vi "Mean Selected.vi"(11 "Mean Data":dbl[](array[numeric])) -> (3 "mean":dbl)   [LabVIEW 2020]
uses:
  <vilib>/Analysis/NI_AALBase.lvlib
  <vilib>/Analysis/baseanly.llb/Mean (DBL).vi
  PCT FGV CMD.ctl
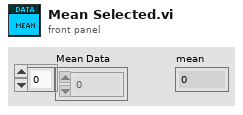
[diagram p1: front panel]
types:
  T1 = typedef "PCT FGV CMD.ctl" = enum16{"INIT", "GET", "SET"}
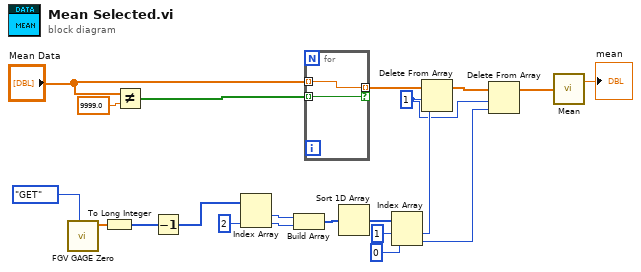
[diagram p0: block diagram]
diagram:
  w3 = 1 ("length")
  n1 = call "FGV GAGE Zero.vi"("CMD"=PCT_FGV_CMD."GET") -> ("output"=w16:dbl[])  [unwired: 9 in, 1 out]
  n2 = To Long Integer(number=w16) -> (32bit integer=w15:i32[])
  n3 = Not Equal?(x="Mean Data", y=9999.0) -> (x != y?=w20:bool[])
  n4 = Decrement(x=w15) -> (x-1=w13:i32[])
  n5 = Index Array(array=w13, index #2=2 ("index")) -> (element #1=w11:i32, element #2=w12:i32)  [unwired: 1 in]
  n6 = Build Array(w11, w12) -> (w10:i32[])
  n7 = for {
    tunnel: "Mean Data" -> [w23] mode=indexing
    tunnel: [w23] -> w21 mode=indexing if=w22
    tunnel: w20 -> [w22] mode=indexing
  }
  n8 = Sort 1D Array(array=w10) -> (sorted array=w8:i32[])
  n9 = Index Array(array=w8, index #1=1 ("index"), index #2=0 ("index")) -> (element #1=w5:i32, element #2=w2:i32)
  n10 = Delete From Array(array=w21, length=w3, index=w5) -> (array with subset deleted=w9:dbl[])  [unwired: 1 out]
  n11 = Delete From Array(array=w9, length=w3, index=w2) -> (array with subset deleted=w4:dbl[])  [unwired: 1 out]
  n12 = call-poly <vilib>:"Mean.vi"("X"=w4) -> ("mean"=→"mean":dbl)  [unwired: 1 out]
